vi "Update Channel Tree by Reference.vi"(7 "Direction to Include":T4, 8 "error in (no error)":errorcluster, 10 "Channnel Tree ref in":refnum<vi>, 11 "Channels":T1[][](array[typedef])) -> (0 "error out":errorcluster, 4 "Update":bool)   [LabVIEW 2021, in "CIF_UI.lvclass"]
uses:
  CIF_UI.lvclass
  CIFCore/Grpc/CIFCoreChannel_client/RPC Messages/cif_management_common_ChannelDirection.ctl
  CIFCore/Grpc/CIFCoreChannel_client/CIFCoreChannel_client.lvlib
  CIFCore/Grpc/CIFCoreChannel_client/RPC Messages/cif_management_common_Channel.ctl
  CIFCore/Common/CIFCoreCommon.lvlib
  CIFCore/Grpc/CIFCoreChannel_client/RPC Messages/cif_management_common_ChannelPattern.ctl
  Typedef/Direction to Include.ctl
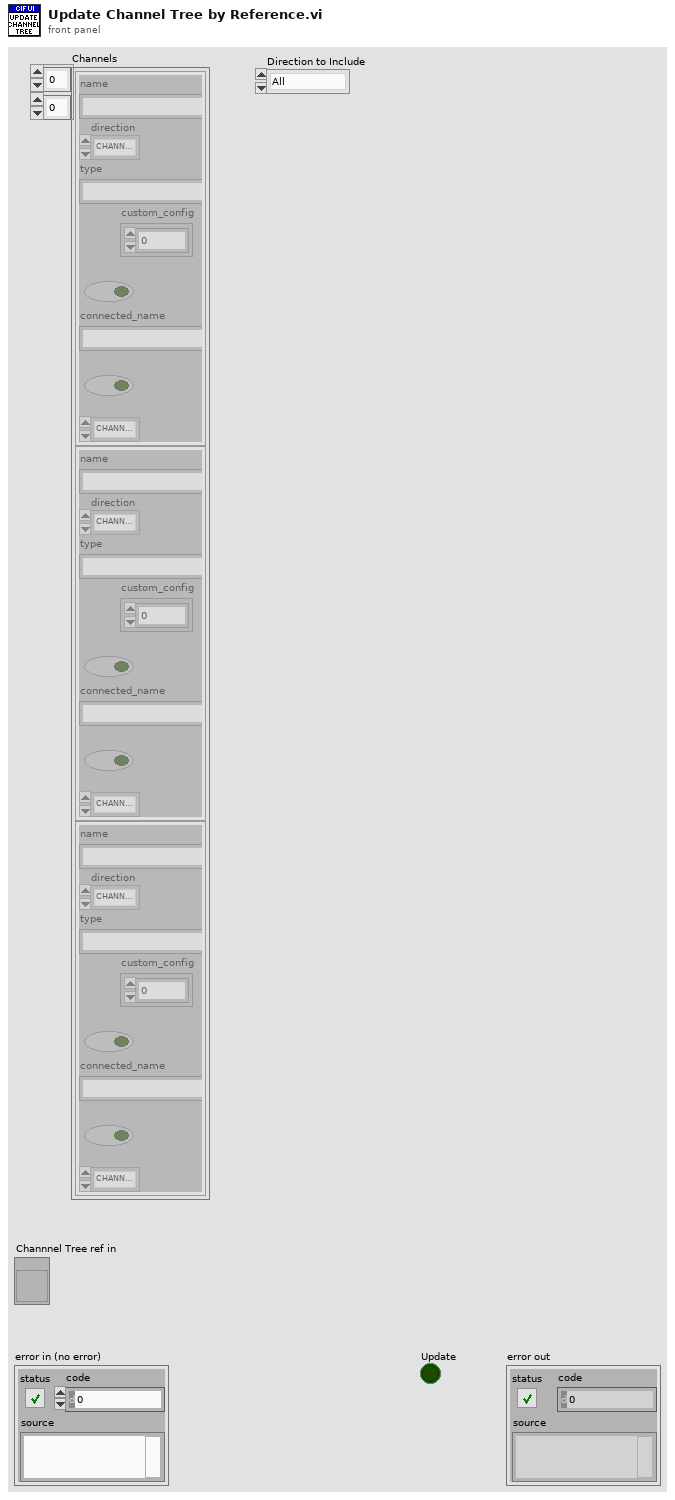
[diagram p1: front panel]
types:
  T1 = typedef "CIFCoreChannel_client.lvlib/cif_management_common_Channel.ctl" = cluster{"name":string, "direction":T2, "type":string, "custom_config":u8[], "connected":bool, "connected_name":string, "forced":bool, "channel_pattern":T3}
  T2 = typedef "CIFCoreChannel_client.lvlib/cif_management_common_ChannelDirection.ctl" = enum32{"CHANNELDIRECTION_UNKNOWN", "CHANNELDIRECTION_PUBLISHER", "CHANNELDIRECTION_SUBSCRIBER"}
  T3 = typedef "CIFCoreChannel_client.lvlib/cif_management_common_ChannelPattern.ctl" = enum32{"CHANNELPATTERN_UNKNOWN", "CHANNELPATTERN_TAG", "CHANNELPATTERN_FIFO", "CHANNELPATTERN_MULTIFIFO", "CHANNELPATTERN_BACKPRESSUREFIFO"}
  T4 = typedef "CIF_UI.lvclass/Direction to Include.ctl" = enum16{"All", "Subscriber", "Publisher"}
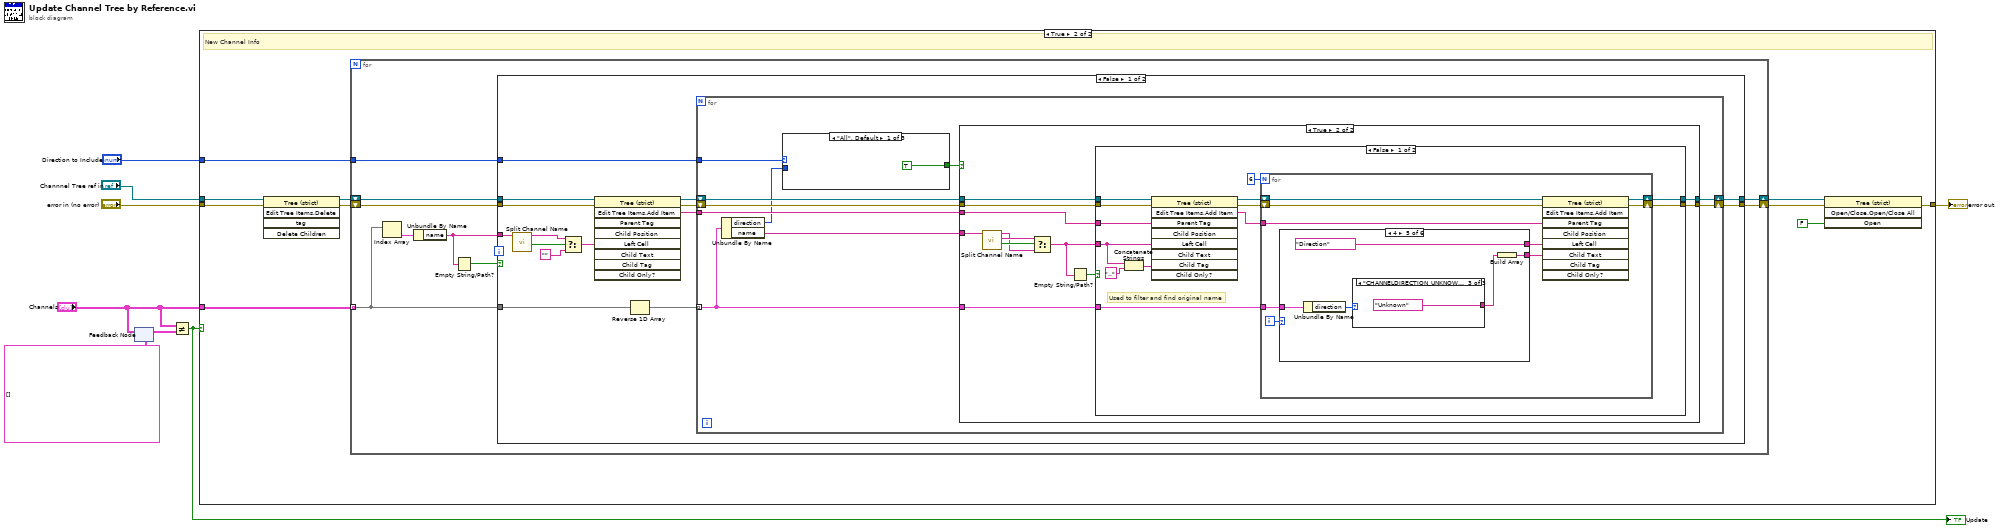
[diagram p0: block diagram]
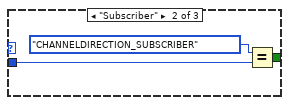
[diagram p3: hidden frame]
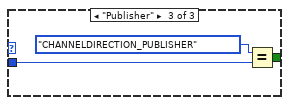
[diagram p4: hidden frame]
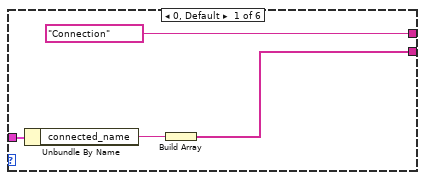
[diagram p6: hidden frame]
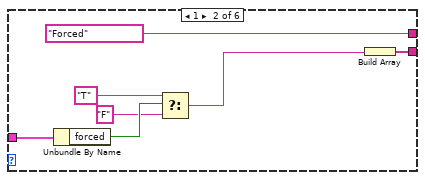
[diagram p7: hidden frame]
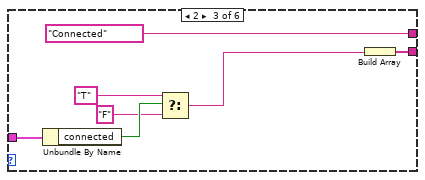
[diagram p8: hidden frame]
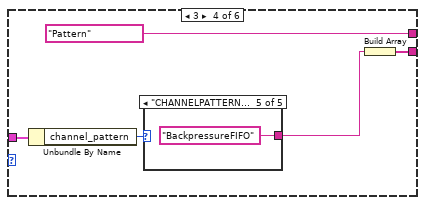
[diagram p9: hidden frame]
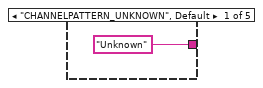
[diagram p10: hidden frame]
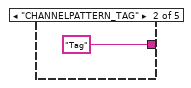
[diagram p11: hidden frame]
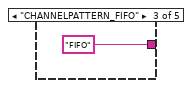
[diagram p12: hidden frame]
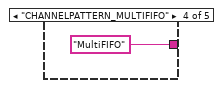
[diagram p13: hidden frame]
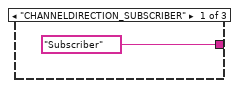
[diagram p14: hidden frame]
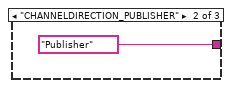
[diagram p15: hidden frame]
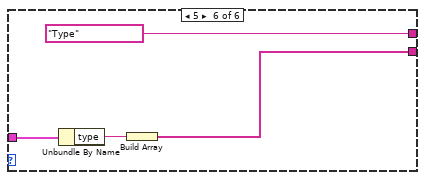
[diagram p16: hidden frame]
diagram:
  n1 = feedback-in #1("Channels") -> ()
  n2 = feedback #1(T1[][] [] ("Channels")) -> (w5:T1[][])
  n3 = Not Equal?(x="Channels", y=w5) -> (x != y?=w4:bool)
  "Update" <- w4
  n4 = case shown="True" w4 {
    tunnel: "error in (no error)" -> [w9 w14]
    tunnel: [w9 w13] -> w7
    tunnel: "Channnel Tree ref in" -> [_ w10]
    tunnel: "Channels" -> [_ w12]
    tunnel: "Direction to Include" -> [_ w11]
    frame False {
      # "No updates"
    }
    frame True {
      # "New Channel Info"
      n5 = invoke class="Tree (strict)" method="Edit Tree Items.Delete"(reference=w10, error in=w14) -> (reference out=w18:refnum<vi>, error out=w19:errorcluster)  [unwired: 3 in, 3 out]
      n6 = for {
        shift-right: [w27] -> w17
        shift-left: w18 -> [w26]
        tunnel: w12 -> [w24] mode=indexing
        tunnel: w11 -> [w22]
        shift-right: [w28] -> w16
        shift-left: w19 -> [w25]
        n7 = Index Array(array=w24) -> (element=w23:T1)  [unwired: 1 in]
        n8 = Unbundle By Name(w23) -> ("name"=w21:string)
        n9 = Empty String/Path?(string/path=w21) -> (empty?=w20:bool)
        n10 = case shown="False" w20 {
          tunnel: [w43 w139] -> w28
          tunnel: [w42 w140] -> w27
          tunnel: w26 -> [w41 w140]
          tunnel: w25 -> [w40 w139]
          tunnel: w24 -> [w39 _]
          tunnel: w22 -> [w38 _]
          tunnel: w21 -> [w33 _]
          frame False {
            n11 = call "Split Channel Name.vi"("Channel Name"=w33) -> ("Split"=w32:bool, "Parent"=w31:string)  [unwired: 8 in, 1 out]
            n12 = Select(t=w31, s=w32, f="") -> (s? t:f=w30:string)
            n13 = invoke class="Tree (strict)" method="Edit Tree Items.Add Item"(reference=w41, error in=w40, "Left Cell"=w30) -> (reference out=w37:refnum<vi>, error out=w36:errorcluster, "Edit Tree Items:Add Item"=w35:string)  [unwired: 6 in, 6 out]
            n14 = Reverse 1D Array(array=w39) -> (reversed array=w34:T1[])
            n15 = for {
              tunnel: w35 -> [w51]
              shift-right: [w49] -> w42
              shift-left: w37 -> [w53]
              shift-right: [w50] -> w43
              shift-left: w36 -> [w52]
              tunnel: w34 -> [w48] mode=indexing
              tunnel: w38 -> [w44]
              n16 = Unbundle By Name(w48) -> ("direction"=w45:T2, "name"=w47:string)
              n17 = case shown="\"All\", Default" w44 {
                tunnel: [TRUE w57 w60] -> w46
                tunnel: w45 -> [_ w56 w59]
                frame "All", Default {
                }
                frame "Subscriber" {
                  n18 = Equal?(x=cif_management_common_ChannelDirection."CHANNELDIRECTION_SUBSCRIBER" ("y"), y=w56) -> (x = y?=w57:bool)
                }
                frame "Publisher" {
                  n19 = Equal?(x=cif_management_common_ChannelDirection."CHANNELDIRECTION_PUBLISHER" ("y"), y=w59) -> (x = y?=w60:bool)
                }
              }
              n20 = case shown="True" w46 {
                tunnel: w53 -> [w62 w74]
                tunnel: w52 -> [w61 w73]
                tunnel: w51 -> [_ w72]
                tunnel: [w61 w71] -> w50
                tunnel: [w62 w70] -> w49
                tunnel: w48 -> [_ w69]
                tunnel: w47 -> [_ w67]
                frame False {
                }
                frame True {
                  n21 = call "Split Channel Name.vi"("Channel Name"=w67) -> ("Split"=w66:bool, "Child"=w65:string, "Parent"=w64:string)  [unwired: 8 in]
                  n22 = Select(t=w65, s=w66, f=w64) -> (s? t:f=w63:string)
                  n23 = Empty String/Path?(string/path=w63) -> (empty?=w68:bool)
                  n24 = case shown="False" w68 {
                    tunnel: w74 -> [w87 w138]
                    tunnel: w73 -> [w86 w137]
                    tunnel: w72 -> [w83 _]
                    tunnel: [w81 w137] -> w71
                    tunnel: [w80 w138] -> w70
                    tunnel: w69 -> [w79 _]
                    tunnel: w63 -> [w77 _]
                    frame False {
                      # "Used to filter and find original name"
                      n25 = Concatenate Strings(w77, "..") -> (w76:string)
                      n26 = invoke class="Tree (strict)" method="Edit Tree Items.Add Item"(reference=w87, error in=w86, "Parent Tag"=w83, "Left Cell"=w77, "Child Tag"=w76) -> (reference out=w85:refnum<vi>, error out=w84:errorcluster, "Edit Tree Items:Add Item"=w82:string)  [unwired: 4 in, 6 out]
                      n27 = for {
                        N: 6 -> [_]
                        tunnel: w82 -> [w94]
                        shift-right: [w92] -> w80
                        shift-left: w85 -> [w96]
                        shift-right: [w93] -> w81
                        shift-left: w84 -> [w95]
                        tunnel: w79 -> [w91]
                        i -> [w90]
                        n28 = case shown="4" w90 {
                          tunnel: w91 -> [w100 w107 w114 w119 w129 w136]
                          tunnel: [w98 w106 w113 w118 w128 w134] -> w89
                          tunnel: ["Connection" "Forced" "Connected" "Pattern" "Direction" "Type"] -> w88
                          frame 0, Default {
                            n29 = Unbundle By Name(w100) -> ("connected_name"=w99:string)
                            n30 = Build Array(w99) -> (w98:string[])
                          }
                          frame 1 {
                            n31 = Unbundle By Name(w107) -> ("forced"=w103:bool)
                            n32 = Select(t="T", s=w103, f="F") -> (s? t:f=w102:string)
                            n33 = Build Array(w102) -> (w106:string[])
                          }
                          frame 2 {
                            n34 = Unbundle By Name(w114) -> ("connected"=w110:bool)
                            n35 = Select(t="T", s=w110, f="F") -> (s? t:f=w109:string)
                            n36 = Build Array(w109) -> (w113:string[])
                          }
                          frame 3 {
                            n37 = Unbundle By Name(w119) -> ("channel_pattern"=w116:T3)
                            n38 = case shown="\"CHANNELPATTERN_BACKPRESSUREFIFO\"" w116 {
                              tunnel: ["Unknown" "Tag" "FIFO" "MultiFIFO" "BackpressureFIFO"] -> w115
                              frame "CHANNELPATTERN_UNKNOWN", Default {
                              }
                              frame "CHANNELPATTERN_TAG" {
                              }
                              frame "CHANNELPATTERN_FIFO" {
                              }
                              frame "CHANNELPATTERN_MULTIFIFO" {
                              }
                              frame "CHANNELPATTERN_BACKPRESSUREFIFO" {
                              }
                            }
                            n39 = Build Array(w115) -> (w118:string[])
                          }
                          frame 4 {
                            n40 = Unbundle By Name(w129) -> ("direction"=w126:T2)
                            n41 = case shown="\"CHANNELDIRECTION_UNKNOWN\"" w126 {
                              tunnel: ["Subscriber" "Publisher" "Unknown"] -> w125
                              frame "CHANNELDIRECTION_SUBSCRIBER" {
                              }
                              frame "CHANNELDIRECTION_PUBLISHER" {
                              }
                              frame "CHANNELDIRECTION_UNKNOWN" {
                              }
                            }
                            n42 = Build Array(w125) -> (w128:string[])
                          }
                          frame 5 {
                            n43 = Unbundle By Name(w136) -> ("type"=w135:string)
                            n44 = Build Array(w135) -> (w134:string[])
                          }
                        }
                        n45 = invoke class="Tree (strict)" method="Edit Tree Items.Add Item"(reference=w96, error in=w95, "Parent Tag"=w94, "Left Cell"=w88, "Child Text"=w89) -> (reference out=w92:refnum<vi>, error out=w93:errorcluster)  [unwired: 4 in, 7 out]
                      }
                    }
                    frame True {
                    }
                  }
                }
              }
            }
          }
          frame True {
          }
        }
      }
      n46 = invoke class="Tree (strict)" method="Open/Close.Open/Close All"(reference=w17, error in=w16, "Open"=FALSE ("Open?")) -> (error out=w13:errorcluster)  [unwired: 1 in, 3 out]
    }
  }
  "error out" <- w7
